vi "Delta measure (SubVI).vi"(5 "change?":bool, 6 "current":dbl, 7 "ch":i32, 8 "错误输入（无错误）":errorcluster, 11 "输出簇 2":T1={"initialize"=enum."SR830", "6221"={"6221 Resource"="GPIB0::24::INSTR", "Delta status"=FALSE, "电流|RMS(A)"=0.0}, "SR830+6221"={"source"=0, "Current(A)"=0.0, "阻抗(Ohm)"=0.0, "SR830 1"=FALSE, "SR830 2"=FALSE, "SR830 3"=FALSE, "SR830 4"=FALSE, "VISA 1"="", "VISA 2"="", "VISA 3"="", "VISA 4"="", "Reserve 1"=0, "Reserve 2"=-1, "Reserve 3"=-1, "Reserve 4"=-1, "Sensitivity 1"=-1, "Sensitivity 2"=0, "Sensitivity 3"=-1, "Sensitivity 4"=-1, "量程入 1"=0, "量程入 2"=0, "量程入 3"=0, "量程入 4"=0}, "2400"={"2400"=FALSE, "VISA"="", "Output Level (0)"=1e-05, "Compliance  Level (0.1)"=10.0}, "ch"={"ch"=[], "current"=[], "change?"=[], "holding current\nwhen change ch?"=FALSE}, "Instrument"={"335 Resource"="GPIB0::24::INSTR", "Input (0:A)"=0, "Instrument Type"=enum."PPMS-Rotate", "quantum design"=refnum, "Heater Output (1:1)"=1, "semaphore"=refnum, "TCP master instance"=refnum, "335 Status"=refnum, "M24C Resource"="GPIB0::24::INSTR", "4G supply"="GPIB0::24::INSTR", "Temp Status 24C"=refnum, "Temp"=refnum, "9T信号"=refnum, "limit"={"Field limit"=0.0, "Field rate limit"=0.0, "Temp limit"=0.0, "Temp low limit"=0.0, "Temp rate limit "=0.0}, "4g supply status"=refnum, "vi路径"="", "325 Resource "="GPIB0::24::INSTR", "Input (0:A) 325"=0, "Input (1;B)"=1, "in-plane"="", "out-plane"="", "in-plane"=FALSE, "out-plane"=FALSE, "in plane 信号"=refnum}, "Aborting"=refnum, "数据文件"=refnum, "warning"=refnum, "2614B"={"2614B chA"=FALSE, "2614B chB"=FALSE, "VISA"=""}, "33522b"={"33522b resource name"="", "零电压"=0.0, "最大电压"=148.0, "间隔"=4.0, "最小电压"=-48.0, "PZT Scan?"=FALSE}, "gating type"=enum."2614(daul)"} {"Instrument"."Input (1;B)" items=["A", "B"]; "Instrument"."Input (0:A) 325" items=["A", "B"]; "Instrument"."Input (0:A)" items=["A", "B"]; "Instrument"."Heater Output (1:1)" items=["1"=1, "2"=2]; "SR830+6221"."Sensitivity 4" items=["Auto Gain"=-1, "2 nV/fA"=0, "5 nV/fA"=1, "10 nV/fA"=2, "20 nV/fA"=3, "50 nV/fA"=4, "100 nV/fA"=5, "200 nV/fA"=6, "500 nV/fA"=7, "1 uV/pA"=8, "2 uV/pA"=9, "5 uV/pA"=10, "10 uV/pA"=11, "20 uV/pA"=12, "50 uV/pA"=13, "100 uV/pA"=14, "200 uV/pA"=15, "500 uV/pA"=16, "1 mV/nA"=17, "2 mV/nA"=18, "5 mV/nA"=19, "10 mV/nA"=20, "20 mV/nA"=21, "50 mV/nA"=22, "100 mV/nA"=23, "200 mV/nA"=24, "500 mV/mA"=25, "1 V/uA"=26]; "SR830+6221"."Sensitivity 3" items=["Auto Gain"=-1, "2 nV/fA"=0, "5 nV/fA"=1, "10 nV/fA"=2, "20 nV/fA"=3, "50 nV/fA"=4, "100 nV/fA"=5, "200 nV/fA"=6, "500 nV/fA"=7, "1 uV/pA"=8, "2 uV/pA"=9, "5 uV/pA"=10, "10 uV/pA"=11, "20 uV/pA"=12, "50 uV/pA"=13, "100 uV/pA"=14, "200 uV/pA"=15, "500 uV/pA"=16, "1 mV/nA"=17, "2 mV/nA"=18, "5 mV/nA"=19, "10 mV/nA"=20, "20 mV/nA"=21, "50 mV/nA"=22, "100 mV/nA"=23, "200 mV/nA"=24, "500 mV/mA"=25, "1 V/uA"=26]; "SR830+6221"."Sensitivity 1" items=["Auto Gain"=-1, "2 nV/fA"=0, "5 nV/fA"=1, "10 nV/fA"=2, "20 nV/fA"=3, "50 nV/fA"=4, "100 nV/fA"=5, "200 nV/fA"=6, "500 nV/fA"=7, "1 uV/pA"=8, "2 uV/pA"=9, "5 uV/pA"=10, "10 uV/pA"=11, "20 uV/pA"=12, "50 uV/pA"=13, "100 uV/pA"=14, "200 uV/pA"=15, "500 uV/pA"=16, "1 mV/nA"=17, "2 mV/nA"=18, "5 mV/nA"=19, "10 mV/nA"=20, "20 mV/nA"=21, "50 mV/nA"=22, "100 mV/nA"=23, "200 mV/nA"=24, "500 mV/mA"=25, "1 V/uA"=26]; "SR830+6221"."Sensitivity 2" items=["Auto Gain"=-1, "2 nV/fA"=0, "5 nV/fA"=1, "10 nV/fA"=2, "20 nV/fA"=3, "50 nV/fA"=4, "100 nV/fA"=5, "200 nV/fA"=6, "500 nV/fA"=7, "1 uV/pA"=8, "2 uV/pA"=9, "5 uV/pA"=10, "10 uV/pA"=11, "20 uV/pA"=12, "50 uV/pA"=13, "100 uV/pA"=14, "200 uV/pA"=15, "500 uV/pA"=16, "1 mV/nA"=17, "2 mV/nA"=18, "5 mV/nA"=19, "10 mV/nA"=20, "20 mV/nA"=21, "50 mV/nA"=22, "100 mV/nA"=23, "200 mV/nA"=24, "500 mV/mA"=25, "1 V/uA"=26]; "SR830+6221"."Reserve 4" items=["Auto Gain"=-1, "2 nV/fA"=0, "5 nV/fA"=1, "10 nV/fA"=2, "20 nV/fA"=3, "50 nV/fA"=4, "100 nV/fA"=5, "200 nV/fA"=6, "500 nV/fA"=7, "1 uV/pA"=8, "2 uV/pA"=9, "5 uV/pA"=10, "10 uV/pA"=11, "20 uV/pA"=12, "50 uV/pA"=13, "100 uV/pA"=14, "200 uV/pA"=15, "500 uV/pA"=16, "1 mV/nA"=17, "2 mV/nA"=18, "5 mV/nA"=19, "10 mV/nA"=20, "20 mV/nA"=21, "50 mV/nA"=22, "100 mV/nA"=23, "200 mV/nA"=24, "500 mV/mA"=25, "1 V/uA"=26]; "SR830+6221"."Reserve 3" items=["Auto Reserve"=-1, "High Reserve"=0, "Normal"=1, "Low Noise"=2]; "SR830+6221"."Reserve 2" items=["Auto Reserve"=-1, "High Reserve"=0, "Normal"=1, "Low Noise"=2]; "SR830+6221"."Reserve 1" items=["Auto Reserve"=-1, "High Reserve"=0, "Normal"=1, "Low Noise"=2]; "SR830+6221"."source" items=["SR830 1", "SR830 2", "SR830 3", "SR830 4"]}) -> (0 "错误输出":errorcluster, 2 "输出簇 3":T1={"initialize"=enum."SR830", "6221"={"6221 Resource"="GPIB0::24::INSTR", "Delta status"=FALSE, "电流|RMS(A)"=0.0}, "SR830+6221"={"source"=0, "Current(A)"=0.0, "阻抗(Ohm)"=0.0, "SR830 1"=FALSE, "SR830 2"=FALSE, "SR830 3"=FALSE, "SR830 4"=FALSE, "VISA 1"="", "VISA 2"="", "VISA 3"="", "VISA 4"="", "Reserve 1"=0, "Reserve 2"=-1, "Reserve 3"=-1, "Reserve 4"=-1, "Sensitivity 1"=-1, "Sensitivity 2"=0, "Sensitivity 3"=-1, "Sensitivity 4"=-1, "量程入 1"=0, "量程入 2"=0, "量程入 3"=0, "量程入 4"=0}, "2400"={"2400"=FALSE, "VISA"="", "Output Level (0)"=1e-05, "Compliance  Level (0.1)"=10.0}, "ch"={"ch"=[], "current"=[], "change?"=[], "holding current\nwhen change ch?"=FALSE}, "Instrument"={"335 Resource"="GPIB0::24::INSTR", "Input (0:A)"=0, "Instrument Type"=enum."PPMS-Rotate", "quantum design"=refnum, "Heater Output (1:1)"=1, "semaphore"=refnum, "TCP master instance"=refnum, "335 Status"=refnum, "M24C Resource"="GPIB0::24::INSTR", "4G supply"="GPIB0::24::INSTR", "Temp Status 24C"=refnum, "Temp"=refnum, "9T信号"=refnum, "limit"={"Field limit"=0.0, "Field rate limit"=0.0, "Temp limit"=0.0, "Temp low limit"=0.0, "Temp rate limit "=0.0}, "4g supply status"=refnum, "vi路径"="", "325 Resource "="GPIB0::24::INSTR", "Input (0:A) 325"=0, "Input (1;B)"=1, "in-plane"="", "out-plane"="", "in-plane"=FALSE, "out-plane"=FALSE, "in plane 信号"=refnum}, "Aborting"=refnum, "数据文件"=refnum, "warning"=refnum, "2614B"={"2614B chA"=FALSE, "2614B chB"=FALSE, "VISA"=""}, "33522b"={"33522b resource name"="", "零电压"=0.0, "最大电压"=148.0, "间隔"=4.0, "最小电压"=-48.0, "PZT Scan?"=FALSE}, "gating type"=enum."2614(daul)"} {"Instrument"."Input (1;B)" items=["A", "B"]; "Instrument"."Input (0:A) 325" items=["A", "B"]; "Instrument"."Input (0:A)" items=["A", "B"]; "Instrument"."Heater Output (1:1)" items=["1"=1, "2"=2]; "SR830+6221"."Sensitivity 4" items=["Auto Gain"=-1, "2 nV/fA"=0, "5 nV/fA"=1, "10 nV/fA"=2, "20 nV/fA"=3, "50 nV/fA"=4, "100 nV/fA"=5, "200 nV/fA"=6, "500 nV/fA"=7, "1 uV/pA"=8, "2 uV/pA"=9, "5 uV/pA"=10, "10 uV/pA"=11, "20 uV/pA"=12, "50 uV/pA"=13, "100 uV/pA"=14, "200 uV/pA"=15, "500 uV/pA"=16, "1 mV/nA"=17, "2 mV/nA"=18, "5 mV/nA"=19, "10 mV/nA"=20, "20 mV/nA"=21, "50 mV/nA"=22, "100 mV/nA"=23, "200 mV/nA"=24, "500 mV/mA"=25, "1 V/uA"=26]; "SR830+6221"."Sensitivity 3" items=["Auto Gain"=-1, "2 nV/fA"=0, "5 nV/fA"=1, "10 nV/fA"=2, "20 nV/fA"=3, "50 nV/fA"=4, "100 nV/fA"=5, "200 nV/fA"=6, "500 nV/fA"=7, "1 uV/pA"=8, "2 uV/pA"=9, "5 uV/pA"=10, "10 uV/pA"=11, "20 uV/pA"=12, "50 uV/pA"=13, "100 uV/pA"=14, "200 uV/pA"=15, "500 uV/pA"=16, "1 mV/nA"=17, "2 mV/nA"=18, "5 mV/nA"=19, "10 mV/nA"=20, "20 mV/nA"=21, "50 mV/nA"=22, "100 mV/nA"=23, "200 mV/nA"=24, "500 mV/mA"=25, "1 V/uA"=26]; "SR830+6221"."Sensitivity 1" items=["Auto Gain"=-1, "2 nV/fA"=0, "5 nV/fA"=1, "10 nV/fA"=2, "20 nV/fA"=3, "50 nV/fA"=4, "100 nV/fA"=5, "200 nV/fA"=6, "500 nV/fA"=7, "1 uV/pA"=8, "2 uV/pA"=9, "5 uV/pA"=10, "10 uV/pA"=11, "20 uV/pA"=12, "50 uV/pA"=13, "100 uV/pA"=14, "200 uV/pA"=15, "500 uV/pA"=16, "1 mV/nA"=17, "2 mV/nA"=18, "5 mV/nA"=19, "10 mV/nA"=20, "20 mV/nA"=21, "50 mV/nA"=22, "100 mV/nA"=23, "200 mV/nA"=24, "500 mV/mA"=25, "1 V/uA"=26]; "SR830+6221"."Sensitivity 2" items=["Auto Gain"=-1, "2 nV/fA"=0, "5 nV/fA"=1, "10 nV/fA"=2, "20 nV/fA"=3, "50 nV/fA"=4, "100 nV/fA"=5, "200 nV/fA"=6, "500 nV/fA"=7, "1 uV/pA"=8, "2 uV/pA"=9, "5 uV/pA"=10, "10 uV/pA"=11, "20 uV/pA"=12, "50 uV/pA"=13, "100 uV/pA"=14, "200 uV/pA"=15, "500 uV/pA"=16, "1 mV/nA"=17, "2 mV/nA"=18, "5 mV/nA"=19, "10 mV/nA"=20, "20 mV/nA"=21, "50 mV/nA"=22, "100 mV/nA"=23, "200 mV/nA"=24, "500 mV/mA"=25, "1 V/uA"=26]; "SR830+6221"."Reserve 4" items=["Auto Gain"=-1, "2 nV/fA"=0, "5 nV/fA"=1, "10 nV/fA"=2, "20 nV/fA"=3, "50 nV/fA"=4, "100 nV/fA"=5, "200 nV/fA"=6, "500 nV/fA"=7, "1 uV/pA"=8, "2 uV/pA"=9, "5 uV/pA"=10, "10 uV/pA"=11, "20 uV/pA"=12, "50 uV/pA"=13, "100 uV/pA"=14, "200 uV/pA"=15, "500 uV/pA"=16, "1 mV/nA"=17, "2 mV/nA"=18, "5 mV/nA"=19, "10 mV/nA"=20, "20 mV/nA"=21, "50 mV/nA"=22, "100 mV/nA"=23, "200 mV/nA"=24, "500 mV/mA"=25, "1 V/uA"=26]; "SR830+6221"."Reserve 3" items=["Auto Reserve"=-1, "High Reserve"=0, "Normal"=1, "Low Noise"=2]; "SR830+6221"."Reserve 2" items=["Auto Reserve"=-1, "High Reserve"=0, "Normal"=1, "Low Noise"=2]; "SR830+6221"."Reserve 1" items=["Auto Reserve"=-1, "High Reserve"=0, "Normal"=1, "Low Noise"=2]; "SR830+6221"."source" items=["SR830 1", "SR830 2", "SR830 3", "SR830 4"]}, 3 "数组":string[](array[string]))   [LabVIEW 2019, in "SubVI.lvlib"]
uses:
  SubVI.lvlib
  ctl/config.ctl
  <vilib>/NI/Modbus Library/API/Master/Modbus Master.lvclass
  ctl/initialize.ctl
  ctl/Instrument.ctl
  ctl/Instrument Type.ctl
  lib/QDInstrument.dll
  ctl/335 state.ctl
  ctl/limit.ctl
  ctl/9T mag field stauts.ctl
  ctl/warning.ctl
  ctl/Gating type.ctl
  lib/Keithley 622x/Configure/Format/Typedefs/KE622x -- Optional Meas Elements.ctl
  <vilib>/Analysis/baseanly.llb/Mean (DBL).vi
  lib/Keithley 622x/Keithley 622x.lvlib
  Get value.lvlib
  <vilib>/Analysis/NI_AALBase.lvlib
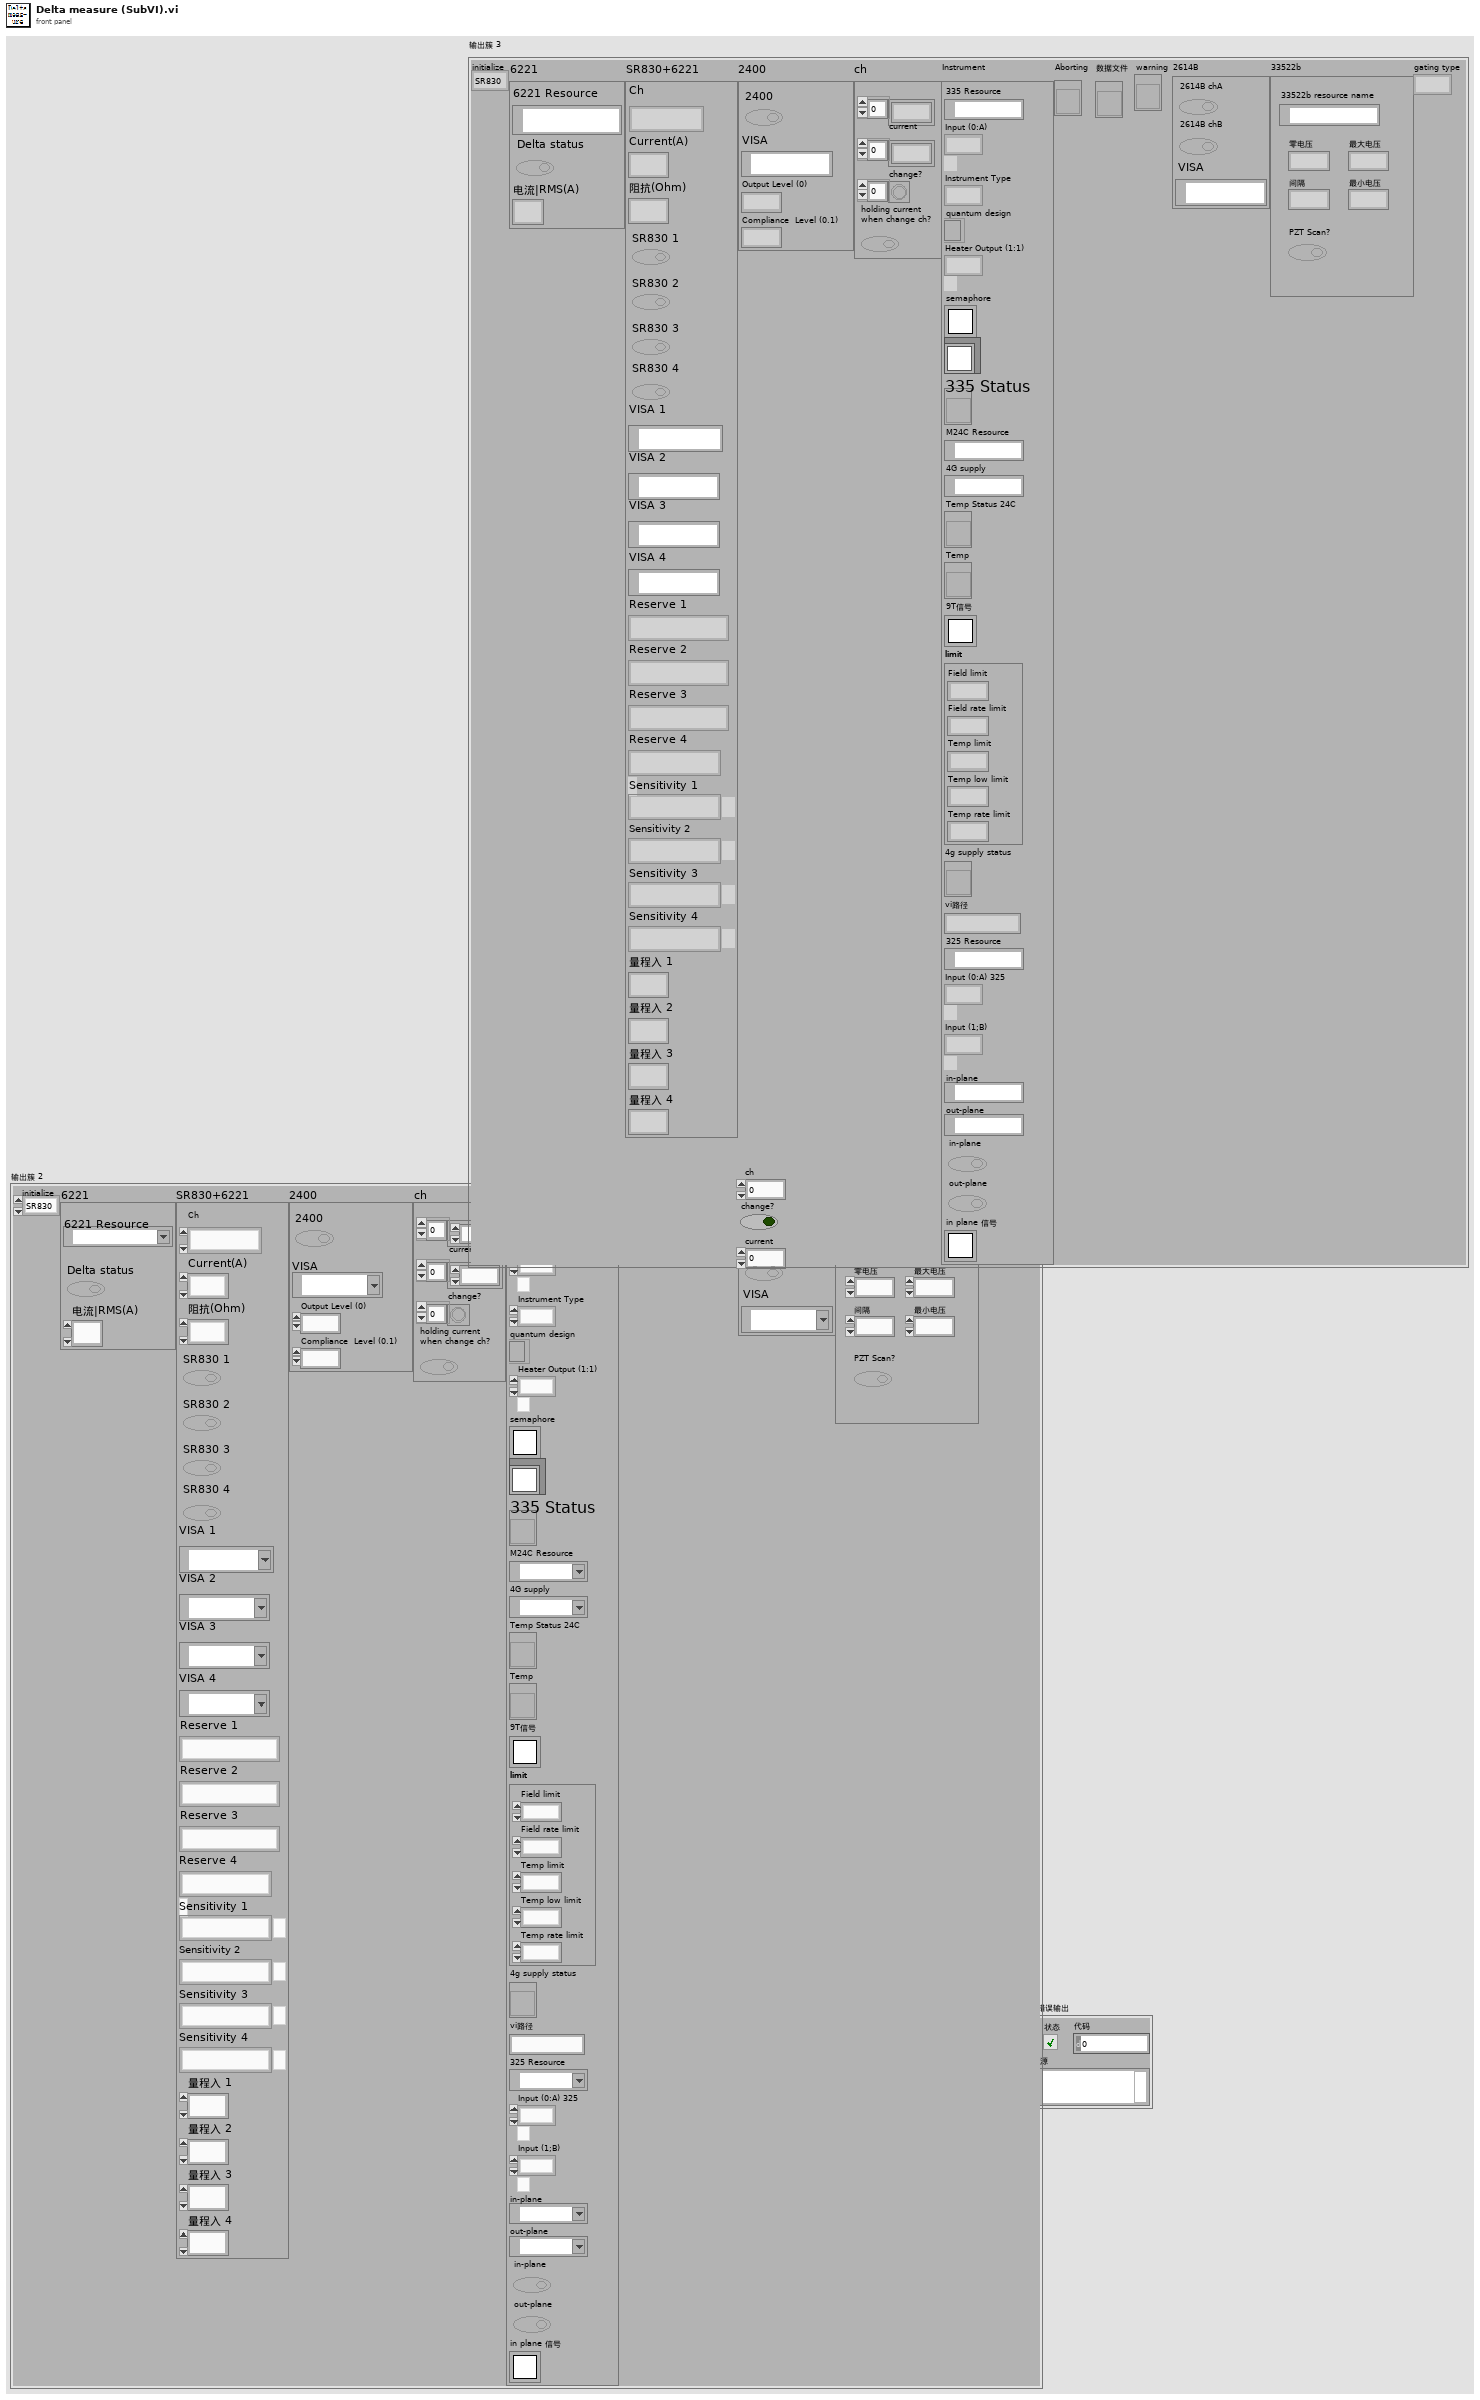
[diagram p1: front panel]
types:
  T1 = typedef "config.ctl" = cluster{"initialize":T2, "6221":cluster{"6221 Resource":refnum<visa-resource-name>, "Delta status":bool, "电流|RMS(A)":dbl}, "SR830+6221":cluster{"source":u16, "Current(A)":dbl, "阻抗(Ohm)":dbl, "SR830 1":bool, "SR830 2":bool, "SR830 3":bool, "SR830 4":bool, "VISA 1":refnum<visa-resource-name>, "VISA 2":refnum<visa-resource-name>, "VISA 3":refnum<visa-resource-name>, "VISA 4":refnum<visa-resource-name>, "Reserve 1":i16, "Reserve 2":i16, "Reserve 3":i16, "Reserve 4":i16, "Sensitivity 1":i16, "Sensitivity 2":i16, "Sensitivity 3":i16, "Sensitivity 4":i16, "量程入 1":i32, "量程入 2":i32, "量程入 3":i32, "量程入 4":i32}, "2400":cluster{"2400":bool, "VISA":refnum<visa-resource-name>, "Output Level (0)":dbl, "Compliance  Level (0.1)":dbl}, "ch":cluster{"ch":i32[], "current":dbl[], "change?":bool[], "holding current\nwhen change ch?":bool}, "Instrument":T3, "Aborting":refnum<vi>, "数据文件":refnum<vi>, "warning":refnum<vi>, "2614B":cluster{"2614B chA":bool, "2614B chB":bool, "VISA":refnum<visa-resource-name>}, "33522b":cluster{"33522b resource name":refnum<visa-resource-name>, "零电压":dbl, "最大电压":dbl, "间隔":dbl, "最小电压":dbl, "PZT Scan?":bool}, "gating type":T7}
  T2 = typedef "initialize.ctl" = enum16{"SR830", "keithley6221-SR830", "Delta", "Delta-tunnelling", "keithley6221-2182-DC", "PZT"}
  T3 = typedef "Instrument.ctl" = cluster{"335 Resource":refnum<visa-resource-name>, "Input (0:A)":u16, "Instrument Type":T4, "quantum design":refnum<k24>, "Heater Output (1:1)":u16, "semaphore":T5, "TCP master instance":refnum<class "Modbus Master.lvclass">, "335 Status":refnum<vi>, "M24C Resource":refnum<visa-resource-name>, "4G supply":refnum<visa-resource-name>, "Temp Status 24C":refnum<vi>, "Temp":refnum<vi>, "9T信号":T5, "limit":T6, "4g supply status":refnum<vi>, "vi路径":string, "325 Resource ":refnum<visa-resource-name>, "Input (0:A) 325":u16, "Input (1;B)":u16, "in-plane":refnum<visa-resource-name>, "out-plane":refnum<visa-resource-name>, "in-plane":bool, "out-plane":bool, "in plane 信号":T5}
  T4 = typedef "Instrument Type.ctl" = enum16{"PPMS", "VersaLab", "DynaCool", "SVSM", "PPMS-Rotate", "Lakeshore335", "9T mag", "test"}
  T5 = typedef "Semaphore RefNum" = refnum<k1>
  T6 = typedef "limit.ctl" = cluster{"Field limit":dbl, "Field rate limit":dbl, "Temp limit":dbl, "Temp low limit":dbl, "Temp rate limit ":dbl}
  T7 = typedef "Gating type.ctl" = enum32{"null", "2614(daul)", "2400"}
  T8 = typedef "Keithley 622x.lvlib/KE622x -- Optional Meas Elements.ctl" = cluster{"Timstamp?":bool, "Reading Num?":bool, "Source Value?":bool, "Compliance?":bool, "Average Voltage?":bool}
  T9 = typedef "Keithley 622x.lvlib/KE622x -- Meas Event Reg State.ctl" = cluster{"B0, ROF:  KE2182A Delta Reading Overflow Event?":bool, "B1, Int:  Interlock OK Event?":bool, "B2, Temp:  Over Temperature Event?":bool, "B3, Comp:  Compliance Event?":bool, "B5, RAV:  Delta Reading Available Event?":bool, "B6, TN:  User Defined Reading Number Stored In Buffer Event?":bool, "B7, BAV:  At Least 2 Readings Stored In Buffer Event?":bool, "B12, BQF:  Buffer Quarter Full Event?":bool, "B8, BHF:  Buffer Half Full Event?":bool, "B13, B3QF:  Buffer 3/4 Full Event?":bool, "B9, BFL:  Buffer Full Event?":bool}
  T10 = typedef "Keithley 622x.lvlib/KE622x -- Trace Buf.ctl" = cluster{"Additional Valid Arrays":T8, "Reading Num":u32[], "Timestamp (secs)":sgl[], "Source Val (A)":sgl[], "Reading":sgl[], "Average Voltage (V)":sgl[], "Compliance?":bool[]}
  T11 = typedef "warning.ctl" = cluster{"Compliance":bool}
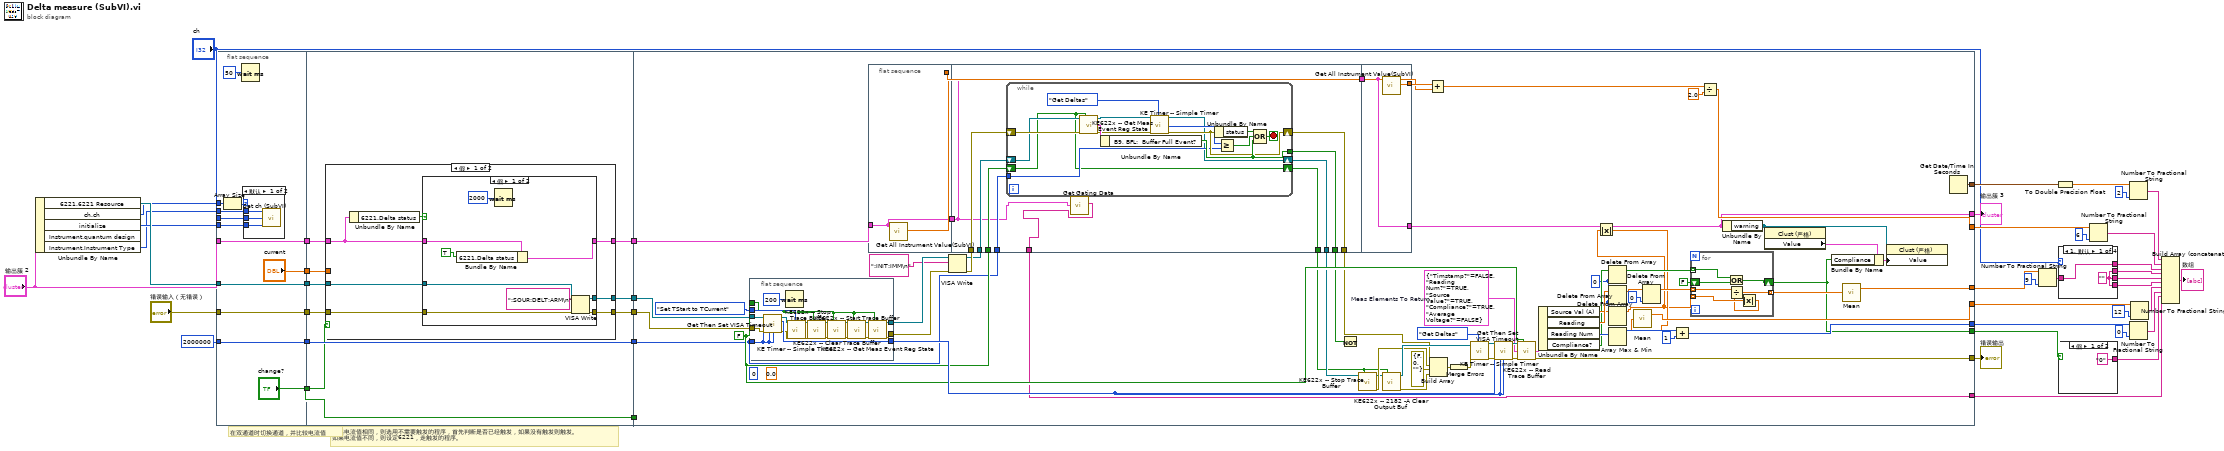
[diagram p0: block diagram]
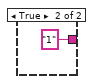
[diagram p2: hidden frame]
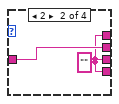
[diagram p3: hidden frame]
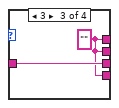
[diagram p4: hidden frame]
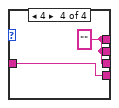
[diagram p5: hidden frame]
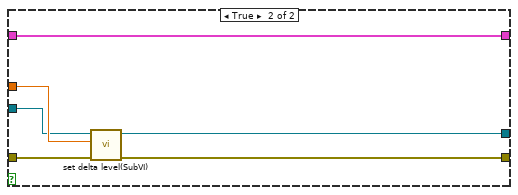
[diagram p8: hidden frame]
diagram:
  # "如果电流值相同，则选用不需要触发的程序，首先判断是否已经触发，如果没有触发则触发。\n如果电流值不同，则设定6221，走触发的程序。"
  # "在双通道时切换通道，并比较电流值"
  n1 = Unbundle By Name("输出簇 2") -> ("6221.6221 Resource"=w31:refnum<visa-resource-name>, "ch.ch"=w7:i32[], "initialize"=w15:T2, "Instrument.Instrument Type"=w6:T4)  [unwired: 1 out]
  n2 = flat-sequence {
    tunnel: u32 2000000 ("Timeout (20000 ms)") -> [w57]
    tunnel: "错误输入（无错误）" -> [w47]
    tunnel: w31 -> [w48]
    tunnel: [w57] -> w45
    tunnel: ["change?"] -> w44
    tunnel: ["current"] -> w43
    tunnel: [w48] -> w42
    tunnel: w15 -> [w51]
    tunnel: "输出簇 2" -> [w56]
    tunnel: [w56] -> w9
    tunnel: w7 -> [w55]
    tunnel: w6 -> [w53]
    tunnel: "ch" -> [w52]
    tunnel: [w47] -> w1
    tunnel: w45 -> [w69]
    tunnel: [w69] -> w41
    tunnel: w44 -> [w64]
    tunnel: w43 -> [w68]
    tunnel: w42 -> [w67]
    tunnel: [w66] -> w40
    tunnel: [w65] -> w39
    tunnel: [w64] -> w38
    tunnel: w9 -> [w63]
    tunnel: [w62] -> w8
    tunnel: w1 -> [w61]
    tunnel: [w132] -> w16
    tunnel: [w101] -> w26
    tunnel: [w133] -> w25
    tunnel: [w100] -> w27
    tunnel: [w140] -> w37
    tunnel: w41 -> [w120]
    tunnel: w40 -> [w139]
    tunnel: w39 -> [w144]
    tunnel: w38 -> [_]
    tunnel: [w128] -> w32
    tunnel: [w98] -> w14
    tunnel: [w95] -> w11
    tunnel: w8 -> [w117]
    tunnel: [w113] -> w5
    frame #0 {
      n3 = Array Size(array=w55) -> (size(s)=w54:i32)
      n4 = Wait (ms)(milliseconds to wait=u32 50) -> ()  [unwired: 1 out]
      n5 = case shown="默认" w54 {
        tunnel: w53 -> [w60 _]
        tunnel: w52 -> [w59 _]
        tunnel: w51 -> [w58 _]
        frame Default {
          n6 = call "Set ch (SubVI).vi"("initialize"=w58, "数值"=w59, "Instrument Type"=w60) -> ()  [unwired: 9 in]
        }
        frame 0, 1 {
        }
      }
    }
    frame #1 {
      n7 = case shown="假" w64 {
        tunnel: w61 -> [w75 w94]
        tunnel: w68 -> [_ w93]
        tunnel: w67 -> [w76 w92]
        tunnel: [w74 w91] -> w65
        tunnel: [w73 w90] -> w66
        tunnel: w63 -> [w71 w89]
        tunnel: [w70 w89] -> w62
        frame False {
          n8 = Unbundle By Name(w71) -> ("6221.Delta status"=w72:bool)
          n9 = case shown="假" w72 {
            tunnel: w76 -> [w81 w87]
            tunnel: [w82 w87] -> w74
            tunnel: w75 -> [w84 w88]
            tunnel: [w83 w88] -> w73
            tunnel: w71 -> [w78 w86]
            tunnel: [w77 w86] -> w70
            frame False {
              n10 = Bundle By Name(cluster=w78, "6221.Delta status"=TRUE) -> (w77:T1)
              n11 = Wait (ms)(milliseconds to wait=u32 2000) -> ()  [unwired: 1 out]
              n12 = VISA Write(VISA resource name=w81, write buffer=":SOUR:DELT:ARM\n" ("format string"), error in (no error)=w84) -> (VISA resource name out=w82:refnum<visa-resource-name>, error out=w83:errorcluster)  [unwired: 1 out]
            }
            frame True {
            }
          }
        }
        frame True {
          n13 = call "set delta level(SubVI).vi"("错误输入（无错误）"=w94, "电流（A）"=w93, "VISA引用句柄输入"=w92) -> ("错误输出"=w90:errorcluster, "VISA引用句柄输出"=w91:refnum<visa-resource-name>)  [unwired: 7 in]
        }
      }
    }
    frame #2 {
      (unwired) 0 ("索引")
      w99 = 0 ("index")
      w125 = FALSE ("Check For SCPI Errors? (T) 2")
      w136 = T8 {"Timstamp?"=FALSE, "Reading Num?"=TRUE, "Source Value?"=TRUE, "Compliance?"=TRUE, "Average Voltage?"=FALSE}  # Meas Elements To Return
      (unwired) sgl 0.0 ("Numeric")
      n14 = flat-sequence {
        tunnel: enum16{"Set TStart to TCurrent", "Get Deltas"}."Set TStart to TCurrent" ("Action") -> [w208]
        tunnel: [w205] -> w153
        tunnel: [w204] -> w152
        tunnel: [w201] -> w145
        tunnel: w144 -> [w198]
        tunnel: w125 -> [w197]
        tunnel: w139 -> [w196]
        tunnel: w120 -> [w195]
        frame #0 {
          n15 = call "Get Then Set VISA Timeout.vi"("VISA Resource Name In"=w198, "New Timeout (msecs)"=w195, "error in (no error)"=w196, "Max Timeout (300 secs)"=w195, "Min Timeout (3 secs)"=w195) -> ("VISA Resource Name Out (dupl)"=w200:refnum<visa-resource-name>, "Old Timeout (msecs)"=w201:u32, "error out"=w199:errorcluster)  [unwired: 7 in, 1 out]
          n16 = Wait (ms)(milliseconds to wait=u32 200) -> ()  [unwired: 1 out]
          n17 = call "KE Timer -- Simple Timer.vi"("Resource In"=w200, "error in (no error)"=w199, "Action"=w208) -> ("Resource Out (dupl)"=w207:refnum<visa-resource-name>, "error out (dupl)"=w206:errorcluster)  [unwired: 7 in, 8 out]
          n18 = call "KE622x -- Stop Trace Buffer.vi"("Resource In"=w207, "Check For SCPI Errors? (T)"=w197, "error in (no error)"=w206) -> ("Resource Out (dupl)"=w212:refnum<visa-resource-name>, "error out"=w211:errorcluster)  [unwired: 11 in]
          n19 = call "KE622x -- Clear Trace Buffer.vi"("Resource In"=w212, "Check For SCPI Errors? (T)"=w197, "error in (no error)"=w211) -> ("Resource Out (dupl)"=w203:refnum<visa-resource-name>, "error out"=w202:errorcluster)  [unwired: 11 in]
          n20 = call "KE622x -- Start Trace Buffer.vi"("Resource In"=w203, "Check For SCPI Errors? (T)"=w197, "error in (no error)"=w202) -> ("Resource Out (dupl)"=w209:refnum<visa-resource-name>, "error out"=w210:errorcluster)  [unwired: 11 in]
          n21 = call "KE622x -- Get Meas Event Reg State.vi"("VISA Resource In"=w209, "Error Query (T)?"=w197, "error in (no error)"=w210) -> ("VISA Resource Out (dupl)"=w205:refnum<visa-resource-name>, "error out"=w204:errorcluster)  [unwired: 10 in, 1 out]
        }
      }
      n22 = flat-sequence {
        tunnel: [w166] -> w118
        tunnel: w117 -> [w165]
        tunnel: [w165] -> w116
        tunnel: w127 -> [w176]
        tunnel: w126 -> [w175]
        tunnel: w125 -> [w174]
        tunnel: [w173] -> w124
        tunnel: [w172] -> w123
        tunnel: [w171] -> w122
        tunnel: [w170] -> w121
        tunnel: w120 -> [w169]
        tunnel: [w167] -> w95
        tunnel: w116 -> [w168]
        tunnel: [w168] -> w115
        tunnel: [w193] -> w119
        tunnel: w115 -> [w192]
        tunnel: [w192] -> w113
        frame #0 {
          n23 = call "Get All Instrument Value(SubVI).vi"("输出簇 2"=w165) -> ("数组"=w166:dbl[])  [unwired: 10 in]
        }
        frame #1 {
          n24 = while {
            shift-right: [w181] -> w173
            shift-left: w176 -> [w191]
            shift-right: [w178] -> w172
            shift-left: w175 -> [w190]
            tunnel: [w183] -> w171
            shift-right: [w177] -> w170
            shift-left: w174 -> [w177]
            tunnel: w169 -> [w179]
            stop <- w184 stop-if-true
            n25 = call "KE622x -- Get Meas Event Reg State.vi"("VISA Resource In"=w190, "Error Query (T)?"=w177, "error in (no error)"=w191) -> ("VISA Resource Out (dupl)"=w187:refnum<visa-resource-name>, "KE622x Meas Event Reg"=w189:T9, "error out"=w188:errorcluster)  [unwired: 10 in]
            n26 = Unbundle By Name(w189) -> ("B9, BFL:  Buffer Full Event?"=w183:bool)
            n27 = call "KE Timer -- Simple Timer.vi"("Resource In"=w187, "error in (no error)"=w188, "Action"=enum16{"Set TStart to TCurrent", "Get Deltas"}."Get Deltas") -> ("Resource Out (dupl)"=w178:refnum<visa-resource-name>, "TCurrent - TStart (ms)"=w185:u32, "error out (dupl)"=w181:errorcluster)  [unwired: 7 in, 7 out]
            n28 = Unbundle By Name(w181) -> ("status"=w180:bool)
            n29 = Greater Or Equal?(x=w185, y=w179) -> (x >= y?=w182:bool)
            n30 = Compound Arithmetic op=OR(w180, w182, w183) -> (w184:bool)
          }
          n31 = call "Get Gating Data.vi"("簇"=w168) -> ("data"=w167:string[])  [unwired: 10 in]
        }
        frame #2 {
          n32 = call "Get All Instrument Value(SubVI).vi"("输出簇 2"=w192) -> ("数组"=w193:dbl[])  [unwired: 10 in]
        }
      }
      n33 = VISA Write(VISA resource name=w153, write buffer=":INIT:IMM\n", error in (no error)=w152) -> (VISA resource name out=w126:refnum<visa-resource-name>, error out=w127:errorcluster)  [unwired: 1 out]
      n34 = Not(x=w122) -> ()  [unwired: 1 out]
      n35 = call "KE622x -- Stop Trace Buffer.vi"("Resource In"=w123, "Check For SCPI Errors? (T)"=w121) -> ("Resource Out (dupl)"=w138:refnum<visa-resource-name>, "error out"=w150:errorcluster)  [unwired: 12 in]
      n36 = call "KE622x -- 2182 -A Clear Output Buf.vi"("622x Resource In"=w138, "Check For SCPI Errors? (T)"=w121) -> ("622x Resource Out (dupl)"=w155:refnum<visa-resource-name>, "error out"=w149:errorcluster)  [unwired: 11 in, 1 out]
      n37 = Add(x=w119, y=w118) -> (x+y=w130:dbl[])
      n38 = Build Array(w124, w150, errorcluster {"status"=FALSE, "code"=0, "source"=""} ("error out"), w149) -> (w151:errorcluster[])
      n39 = Merge Errors(w151) -> (w148:errorcluster)
      n40 = call "KE Timer -- Simple Timer.vi"("Resource In"=w155, "error in (no error)"=w148, "Action"=enum16{"Set TStart to TCurrent", "Get Deltas"}."Get Deltas") -> ("Resource Out (dupl)"=w146:refnum<visa-resource-name>, "error out (dupl)"=w147:errorcluster)  [unwired: 7 in, 8 out]
      n41 = call "Get Then Set VISA Timeout.vi"("VISA Resource Name In"=w146, "New Timeout (msecs)"=w145, "error in (no error)"=w147, "Max Timeout (300 secs)"=w145, "Min Timeout (3 secs)"=w145) -> ("VISA Resource Name Out (dupl)"=w143:refnum<visa-resource-name>, "error out"=w142:errorcluster)  [unwired: 7 in, 2 out]
      n42 = call "KE622x -- Read Trace Buffer.vi"("Resource In"=w143, "Check For SCPI Errors? (T)"=w125, "Meas Elements To Return"=w136, "error in (no error)"=w142) -> ("Trace Buf"=w157:T10, "error out"=w140:errorcluster)  [unwired: 9 in, 1 out]
      n43 = Unbundle By Name(w157) -> ("Source Val (A)"=w107:sgl[], "Reading"=w109:sgl[], "Reading Num"=w141:u32[], "Compliance?"=w106:bool[])
      n44 = Delete From Array(array=w106, index=w99) -> (array with subset deleted=w105:bool[])  [unwired: 1 in, 1 out]
      n45 = Delete From Array(array=w109, index=w99) -> (array with subset deleted=w108:sgl[])  [unwired: 1 in, 1 out]
      n46 = Delete From Array(array=w107, index=w99) -> (array with subset deleted=w96:sgl[])  [unwired: 1 in, 1 out]
      n47 = Absolute Value(x=w96) -> (abs(x)=w97:sgl[])
      n48 = Array Max & Min(array=w141) -> (max value=w135:u32)  [unwired: 3 out]
      n49 = call-poly <vilib>:"Mean.vi"("X"=w97) -> ("mean"=w100:dbl)  [unwired: 1 out]
      n50 = Delete From Array(array=w108, index=0 ("索引")) -> (array with subset deleted=w103:sgl[])  [unwired: 1 in, 1 out]
      n51 = Add(x=w135, y=u32 1) -> (x+y=w133:u32)
      n52 = for {
        tunnel: w105 -> [w164] mode=indexing
        shift-right: [w162] -> w98
        shift-left: FALSE -> [w163]
        tunnel: w96 -> [w159] mode=indexing
        tunnel: w103 -> [w161] mode=indexing
        tunnel: [w160] -> w102 mode=indexing
        n53 = Or(x=w164, y=w163) -> (x .or. y?=w162:bool)
        n54 = Absolute Value(x=w159) -> (abs(x)=w158:sgl)
        n55 = Divide(x=w161, y=w158) -> (x/y=w160:sgl)
      }
      n56 = Divide(x=w130, y=2.0) -> (x/y=w128:dbl[])
      n57 = Unbundle By Name(w113) -> ("warning"=w112:refnum<vi>)
      n58 = property class="Clust (严格)"(reference=w112) -> ("Value"=w111:T11)  [unwired: 1 in, 2 out]
      n59 = Bundle By Name(cluster=w111, "Compliance"=w98) -> (w110:T11)
      n60 = call-poly <vilib>:"Mean.vi"("X"=w102) -> ("mean"=w101:dbl)  [unwired: 1 out]
      n61 = property class="Clust (严格)"(reference=w112, "Value"=w110) -> ()  [unwired: 1 in, 2 out]
      n62 = Get Date/Time In Seconds() -> (seconds since 1Jan1904=w132:timestamp)
    }
  }
  n63 = Number To Fractional String(number=w26, precision (6)=i16 9 ("精度(6)")) -> (F-format string=w21:string)  [unwired: 2 in]
  n64 = To Double Precision Float(number=w16) -> (double precision float=w17:dbl)
  n65 = case shown="1, 默认" "ch" {
    tunnel: w21 -> [w214 w216 w218 w220]
    tunnel: [w214 w215 w217 w219] -> w22
    tunnel: [w213 w216 w217 w219] -> w23
    tunnel: [w213 w215 w218 w219] -> w3
    tunnel: [w213 w215 w217 w220] -> w2
    frame 1, Default {
      w213 = ""
    }
    frame 2 {
      w215 = ""
    }
    frame 3 {
      w217 = ""
    }
    frame 4 {
      w219 = ""
    }
  }
  n66 = case shown="假" w14 {
    tunnel: ["0" "1"] -> w12
    frame False {
    }
    frame True {
    }
  }
  n67 = Number To Fractional String(number=w32, precision (6)=i16 6 ("精度(6)")) -> (F-format string=w13:string[])  [unwired: 2 in]
  n68 = Number To Fractional String(number=w17, precision (6)=i16 2 ("精度(6)")) -> (F-format string=w19:string)  [unwired: 2 in]
  n69 = Number To Fractional String(number=w25, precision (6)=i16 0 ("精度(6)")) -> (F-format string=w29:string)  [unwired: 2 in]
  n70 = Number To Fractional String(number=w27, precision (6)=i16 12) -> (F-format string=w30:string)  [unwired: 2 in]
  n71 = Build Array (concatenate)(w19, w13, w22, w23, w3, w2, w30, w29, w12, w11) -> (→"数组":string[])
  "错误输出" <- w37
  "输出簇 3" <- w5
